vi "Set Color Msg.vi"(8 "error in (no error)":errorcluster, 11 "[V] Main UI in":refnum<class "[V] Main UI.lvclass">) -> (0 "error out":errorcluster, 3 "[V] Main UI out":refnum<class "[V] Main UI.lvclass">)   [LabVIEW 2020, in "[V] Main UI.lvlib" / "[V] Main UI.lvclass"]
uses:
  [V] Main UI.lvclass
  Color Interface/Color/Color Message.lvclass
  MVVM Framework/MVVM Abstruct View/MVVM Abstruct View/MVVM Abstruct View.lvclass/MVVM Abstruct View.ctl
  Color Interface/Color/Color Message.lvclass/Color Message.ctl
  Color Interface/Color Interface Messages/Set Color Msg/Set Color Msg.lvclass/Set Color Msg.ctl
  <vilib>/ActorFramework/Message Enqueuer/Message Enqueuer.lvclass/Message Enqueuer.ctl
  Color Interface/Color/Accessors/Write BG Color.vi
  Color Interface/Color/Accessors/Write txt Color.vi
  MVVM Framework/MVVM Abstruct View/MVVM Abstruct View/Accessor/Read ActorMap-Views.vi
  <vilib>/ActorFramework/Message Enqueuer/Enqueue.vi
  Color Interface/Color Interface Messages/Set Color Msg/Set Color Msg.lvclass
  C:/Program Files (x86)/National Instruments/LabVIEW 2020/vi.lib/ActorFramework/Message/Message.lvclass
  <vilib>/ActorFramework/Message Priority Queue/Priority Enqueue.vi
  Depden On/ActorMap/ActorMap.lvclass
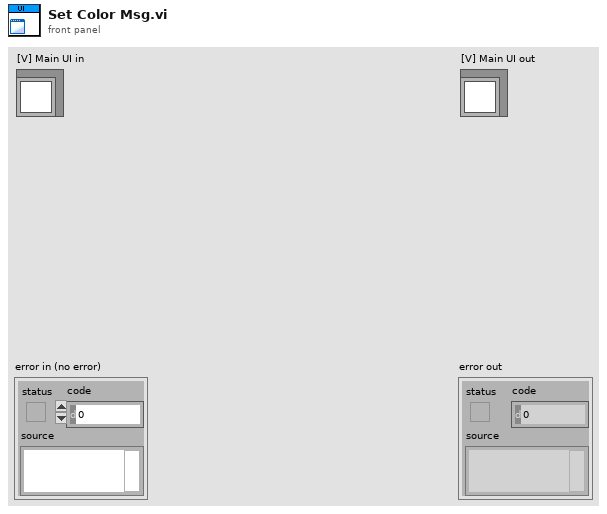
[diagram p1: front panel]
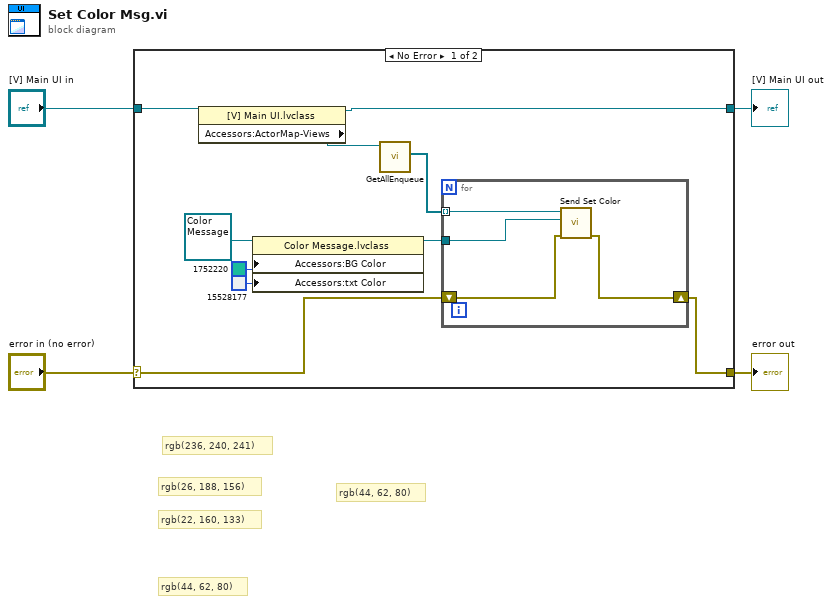
[diagram p0: block diagram]
diagram:
  # "rgb(44, 62, 80)"
  # "rgb(44, 62, 80)"
  # "rgb(22, 160, 133)"
  # "rgb(26, 188, 156)"
  # "rgb(236, 240, 241)"
  n1 = case shown="No Error" "error in (no error)" {
    selector: "error in (no error)" -> [w6 w20]
    tunnel: [w5 w20] -> w3
    tunnel: [w7 w19] -> w1
    tunnel: "[V] Main UI in" -> [w9 w19]
    frame No Error {
      n2 = property class="[V] Main UI.lvclass"(reference=w9) -> (reference out=w7:refnum<class "[V] Main UI.lvclass">, "Accessors:ActorMap-Views"=w8:refnum<class "ActorMap.lvclass">)  [unwired: 1 in, 1 out]
      n3 = property class="Color Message.lvclass"(reference=refnum<class "Color Message.lvclass"> refnum ("Color Message.lvclass"), "Accessors:BG Color"=u32 1752220 ("BG Color"), "Accessors:txt Color"=u32 15528177 ("txt Color")) -> (reference out=w12:refnum<class "Color Message.lvclass">)  [unwired: 1 in, 1 out]
      n4 = call "GetAllEnqueue.vi"("ActorMap in"=w8) -> ("Enqueues"=w14:refnum<class "Message Enqueuer.lvclass">[])  [unwired: 7 in, 3 out]
      n5 = for {
        tunnel: w14 -> [w18] mode=indexing
        tunnel: w12 -> [w17]
        shift-right: [w15] -> w5
        shift-left: w6 -> [w16]
        n6 = call "Send Set Color.vi"("error in (no error)"=w16, "Color Message.lvclass"=w17, "Message Enqueuer"=w18) -> ("error out"=w15:errorcluster)  [unwired: 7 in, 1 out]
      }
    }
    frame Error {
    }
  }
  "error out" <- w3
  "[V] Main UI out" <- w1
